vi "Log Data.vi"(8 "error in (no error)":errorcluster, 9 "Samples to Save In":u32, 10 "Data":waveform(dbl)[](array[waveform]), 11 "Logging Configuration":T1) -> (0 "error out":errorcluster, 1 "Samples to Save Out":u32)   [LabVIEW 2016, in "Logging.lvlib"]
doc: "Use the Write To Measurement File Express VI to log data to disk in a LVM file."
uses:
  Logging.lvlib
  Logging Configuration.ctl
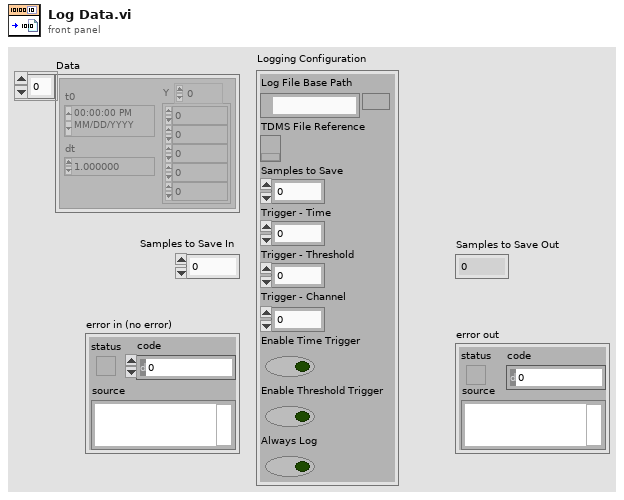
[diagram p1: front panel]
types:
  T1 = typedef "Logging.lvlib/Logging Configuration.ctl" = cluster{"Log File Base Path":path, "TDMS File Reference":refnum<k34>, "Samples to Save":u32, "Trigger - Time":u32, "Trigger - Threshold":dbl, "Trigger - Channel":u32, "Enable Time Trigger":bool, "Enable Threshold Trigger":bool, "Always Log":bool}
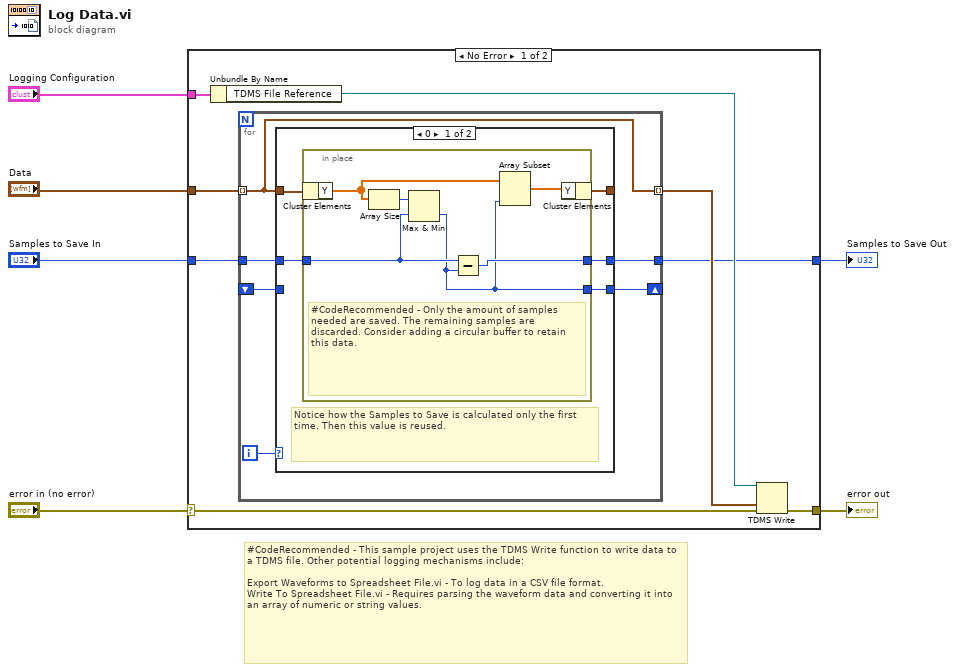
[diagram p0: block diagram]
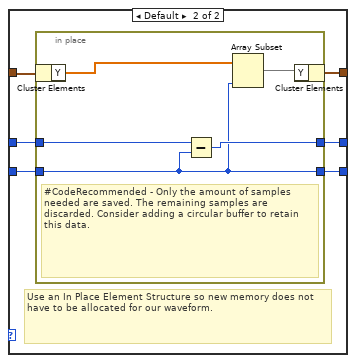
[diagram p2: hidden frame]
diagram:
  # "#CodeRecommended - This sample project uses the TDMS Write function to write data to a TDMS file. Other potential logging mechanisms include:\n\nExport Waveforms to Spreadsheet File.vi - To log data in a CSV file format.\nWrite To Spreadsheet File.vi - Requires parsing the waveform data and converting it into an array of numeric or string values."
  n1 = case shown="No Error" "error in (no error)" {
    selector: "error in (no error)" -> [w11 w44]
    tunnel: "Logging Configuration" -> [w14 _]
    tunnel: "Data" -> [w10 _]
    tunnel: [w12 w44] -> w5
    tunnel: "Samples to Save In" -> [w9 w43]
    tunnel: [w7 w43] -> w1
    frame No Error {
      n2 = Unbundle By Name(w14) -> ("TDMS File Reference"=w13:refnum<k34>)
      n3 = for {
        tunnel: w10 -> [w15] mode=indexing
        tunnel: w9 -> [w20]
        tunnel: [w15] -> w8 mode=indexing
        tunnel: [w19] -> w7
        shift-right: [w17] -> _
        shift-left: _ -> [w16]
        i -> [w18]
        n4 = case shown="0" w18 {
          tunnel: w20 -> [w25 w37]
          tunnel: w15 -> [w21 w33]
          tunnel: [w22 w32] -> _
          tunnel: [w24 w36] -> w19
          tunnel: [w23 w34] -> w17
          tunnel: w16 -> [_ w35]
          frame 0 {
            # "Notice how the Samples to Save is calculated only the first time. Then this value is reused."
            n5 = in-place {
              in-place-border: w25 -> [w30]
              in-place-border: [w29] -> w24
              in-place-border: [w26] -> w23
              # "#CodeRecommended - Only the amount of samples needed are saved. The remaining samples are discarded. Consider adding a circular buffer to retain this data."
              n6 = in-place-cluster #1(w21) -> ("Y"=w28:dbl[])
              n7 = Array Size(array=w28) -> (size(s)=w31:i32)
              n8 = Max & Min(x=w31, y=w30) -> (min(x,y)=w26:u32)  [unwired: 1 out]
              n9 = Subtract(x=w30, y=w26) -> (x-y=w29:u32)
              n10 = Array Subset(array=w28, length=w26) -> (w27:dbl[])  [unwired: 1 in]
              n11 = in-place-cluster #1("Y"=w27) -> (w22:waveform(dbl))
            }
          }
          frame Default {
            # "Use an In Place Element Structure so new memory does not have to be allocated for our waveform."
            n12 = in-place {
              in-place-border: w37 -> [w42]
              in-place-border: [w41] -> w36
              in-place-border: [w38] -> w34
              in-place-border: w35 -> [w38]
              # "#CodeRecommended - Only the amount of samples needed are saved. The remaining samples are discarded. Consider adding a circular buffer to retain this data."
              n13 = in-place-cluster #2(w33) -> ("Y"=w40:dbl[])
              n14 = Subtract(x=w42, y=w38) -> (x-y=w41:u32)
              n15 = Array Subset(array=w40, length=w38) -> (w39:dbl[])  [unwired: 1 in]
              n16 = in-place-cluster #2("Y"=w39) -> (w32:waveform(dbl))
            }
          }
        }
      }
      n17 = TDMS Write(0:w13, 9:w8, 11:w11) -> (15:w12:errorcluster)  [unwired: 3 in, 3 out]
    }
    frame Error {
    }
  }
  "error out" <- w5
  "Samples to Save Out" <- w1
